vi "Protocol.Read Incoming Messages.vi"(8 "error in (no error)":errorcluster, 11 "J1939 Main Configuration":T1) -> (0 "error out":errorcluster)   [LabVIEW 2015, in "J1939 Addon Engine.lvlib"]
uses:
  J1939 Addon Engine.lvlib
  Types/Protocol.Configuration.ctl
  <vilib>/NI/NIVS Addon Network Comm/Engine/VeriStand Comm.lvclass
  <vilib>/NI/NIVS Inline Async API/_VS Inline Async API/Process/Process.lvclass
  Types/Protocol.Refs.ctl
  Shared/J1939 Utilities/Types/CAN Outgoing Message Cluster.ctl
  Types/Protocol.RQST Lookup Table Reference.ctl
  Types/Protocol.Address Table Reference.ctl
  Types/Protocol.XNET Settings.ctl
  Types/Protocol.RQST Lookup Table Action.ctl
  <vilib>/NI/NIVS Inline Async API/_VS Inline Async API/Process/Process.lvclass/Process.ctl
  Protocol.Filter by Device Address.vi
  Protocol.Process Incoming Messages by PDU F.vi
  <vilib>/NI/NIVS Inline Async API/_VS Inline Async API/Error Handling Process/SubVIs/Error.ConvertArray.vi
  Protocol.Parse Message Type.vi
  Shared/J1939 Utilities/Common Conversions.vi
  Shared/J1939 Utilities/SubVIs/Convert CAN Arb ID to J1939 ID.vi
  Protocol.RQST Look for Response.vi
  Shared/J1939 Utilities/SubVIs/Convert J1939 ID to CAN Arb ID.vi
  Shared/J1939 Utilities/SubVIs/Convert CAN Data (U32) to U8.vi
  Protocol.Get Simulated Previously Active DTCs.vi
  Protocol.Get Simulated Active DTCs.vi
  Shared/J1939 Utilities/Common Messages.vi
  Shared/J1939 Utilities/SubVIs/Acknowledgement.vi
  Protocol.Send Reset Previously Active DTC to Main.vi
  Protocol.Send Reset Active DTC to Main.vi
  Protocol.Convert Signals to Frame by ID.vi
  Protocol.Address Lookup Table Action.vi
  Protocol.Convert Data to DTC Frame.vi
  Protocol.Address Lookup Table.vi
  <vilib>/xnet/xnet.llb/XNET Clear.vi
  <vilib>/xnet/xnet.llb/XNET Convert.vi
  <vilib>/xnet/xnet.llb/XNET Convert (Signal to Frame CAN).vi
  <vilib>/xnet/xnet.llb/XNET Create Session.vi
  <vilib>/xnet/xnet.llb/XNET Create Session (Conversion).vi
  Protocol.RQST Lookup Table.vi
  <vilib>/xnet/xnet.llb/XNET Read (Frame CAN).vi
  Shared/J1939 Utilities/J1939 Utilities.lvlib
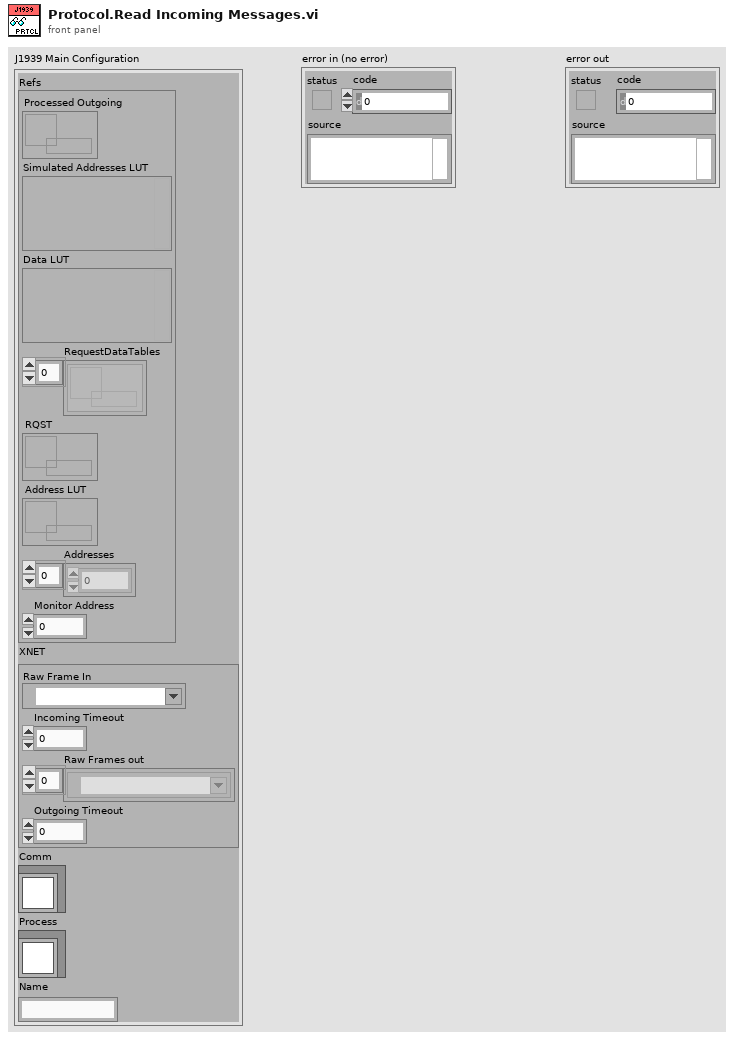
[diagram p1: front panel]
types:
  T1 = typedef "J1939 Addon Engine.lvlib/Protocol.Configuration.ctl" = cluster{"Refs":T2, "XNET":T5, "Comm":refnum<class "VeriStand Comm.lvclass">, "Process":refnum<class "Process.lvclass">, "Name":string}
  T2 = typedef "J1939 Addon Engine.lvlib/Protocol.Refs.ctl" = cluster{"Processed Outgoing":refnum<queue>, "Simulated Addresses LUT":variant, "Data LUT":variant, "RequestDataTables":refnum<k33>[], "RQST":T3, "Address LUT":T4, "Addresses":u8[], "Monitor Address":u8}
  T3 = typedef "J1939 Addon Engine.lvlib/Protocol.RQST Lookup Table Reference.ctl" = refnum<data-value>
  T4 = typedef "J1939 Addon Engine.lvlib/Protocol.Address Table Reference.ctl" = refnum<data-value>
  T5 = typedef "J1939 Addon Engine.lvlib/Protocol.XNET Settings.ctl" = cluster{"Raw Frame In":refnum<k21>, "Incoming Timeout":u32, "Raw Frames out":refnum<k21>[], "Outgoing Timeout":u32}
  T6 = typedef "J1939 Addon Engine.lvlib/Protocol.RQST Lookup Table Action.ctl" = enum16{"Initialize", "Add", "Get", "Remove", "Get Active Requests"}
  T7 = typedef "XNET Frame CAN.ctl" = cluster{"timestamp":timestamp, "payload":u8[], "identifier":u32, "type":T8, "extended?":bool, "echo?":bool}
  T8 = typedef "XNET Frame Type CAN.ctl" = u8
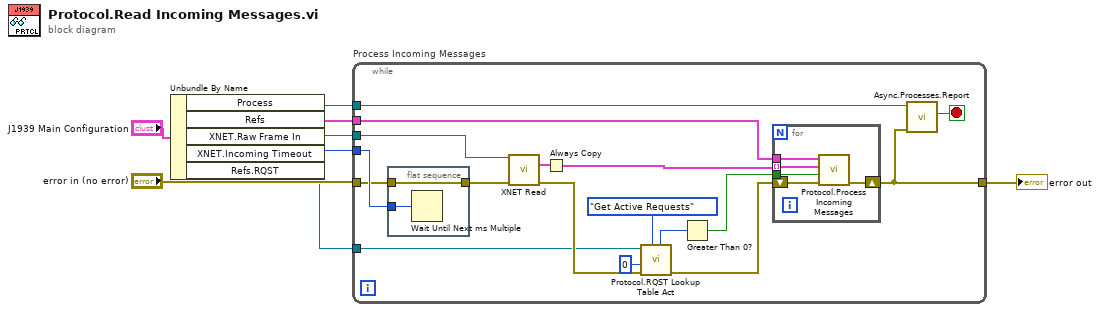
[diagram p0: block diagram]
diagram:
  n1 = Unbundle By Name("J1939 Main Configuration") -> ("Process"=w5:refnum<class "Process.lvclass">, "Refs"=w2:T2, "XNET.Raw Frame In"=w6:refnum<k21>, "XNET.Incoming Timeout"=w7:u32, "Refs.RQST"=w1:T3)
  n2 = while "Process Incoming Messages" {
    tunnel: w2 -> [w25]
    tunnel: "error in (no error)" -> [w15]
    tunnel: [w11] -> w3
    tunnel: w6 -> [w24]
    tunnel: w5 -> [w13]
    tunnel: w7 -> [w22]
    tunnel: w1 -> [w14]
    stop <- w12 stop-if-true
    n3 = flat-sequence {
      tunnel: w22 -> [w27]
      tunnel: [w26] -> w16
      tunnel: w15 -> [w26]
      frame #0 {
        n4 = Wait Until Next ms Multiple(millisecond multiple=w27) -> ()  [unwired: 1 out]
      }
    }
    n5 = call-poly <vilib>:"XNET Read.vi"("session in"=w24, "error in (no error)"=w16) -> ("data"=w23:T7[], "error out"=w19:errorcluster)  [unwired: 12 out]
    n6 = Always Copy(1:w23) -> (0:w21:T7[])
    n7 = call "Protocol.RQST Lookup Table Act.vi"("Action"=Protocol.RQST_Lookup_Table_Action."Get Active Requests", "error in (no error)"=w19, "ID"=u32 0, "Rqst LUT"=w14) -> ("error out"=w18:errorcluster, "# of Active Requests"=w9:i32)  [unwired: 3 in, 3 out]
    n8 = Greater Than 0?(x=w9) -> (x > 0?=w17:bool)
    n9 = for {
      tunnel: w21 -> [w32] mode=indexing
      shift-right: [w30] -> w11
      shift-left: w18 -> [w31]
      tunnel: w25 -> [w29]
      tunnel: w17 -> [w28]
      n10 = call "Protocol.Process Incoming Messages.vi"("error in"=w31, "Active Request?"=w28, "CAN frame"=w32, "J1939 Cluster"=w29) -> ("error out"=w30:errorcluster)  [unwired: 6 in, 1 out]
    }
    n11 = call <vilib>:"Async.Processes.Report.vi"("Error"=w11, "Process in"=w13) -> ("Stop"=w12:bool)  [unwired: 8 in, 1 out]
  }
  "error out" <- w3
